vi "Load and Validate.vi"(8 "error in (no error)":errorcluster, 10 "Report Folder":path, 11 "Project Path":path) -> (0 "error out":errorcluster, 1 "Valid?":bool, 2 "Invalid Sections":string[](array[string]), 3 "Run cluster":T1)   [LabVIEW 2020, in "ProjectBuilder.lvlib" / "Project Builder.lvclass"]
uses:
  Project Builder.lvclass
  Ctl/Ctl_Run Cluster.ctl
  Action/Project Action/Project Action.lvclass
  Report Action/Report Action/Report Action.lvclass
  Ctl/Ctl_Build Steps.ctl
  Action/Project Action/Project Action.lvclass/Project Action.ctl
  PPL/HDH.ClassLoader.lvlibp
  <vilib>/Utility/config.llb/NI_LVConfig.lvlib
  ProjectBuilder.lvlib
  <vilib>/Utility/Data Type/NI_Data Type.lvlib
  Interface/Action Interface/Action Interface.lvclass
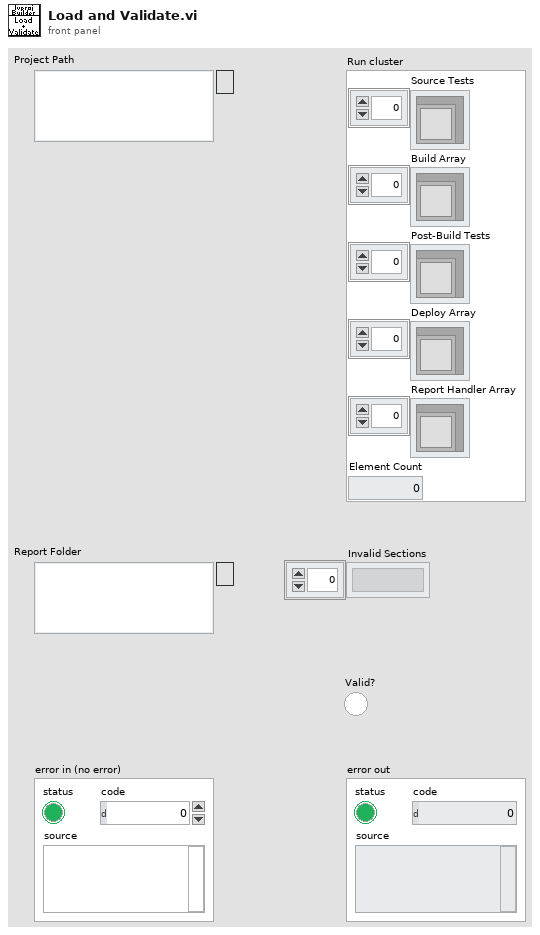
[diagram p1: front panel]
types:
  T1 = typedef "ProjectBuilder.lvlib/Project Builder.lvclass/Ctl_Run Cluster.ctl" = cluster{"Source Tests":refnum<class "Project Action.lvclass">[], "Build Array":refnum<class "Project Action.lvclass">[], "Post-Build Tests":refnum<class "Project Action.lvclass">[], "Deploy Array":refnum<class "Project Action.lvclass">[], "Report Handler Array":refnum<class "Report Action.lvclass">[], "Element Count":i32}
  T2 = typedef "ProjectBuilder.lvlib/Ctl_Build Steps.ctl" = enum16{"Source Test", "Build", "Post-Build Test", "Deploy", "Report"}
  T3 = typedef "NI_LVConfig.lvlib/Config Data RefNum.ctl" = refnum<k1>
  T4 = cluster{"Build Step":T2, "Last number":i32, "String":string}
  T5 = cluster{"Build Step":T2, "Last number":i32, "String":string}[]
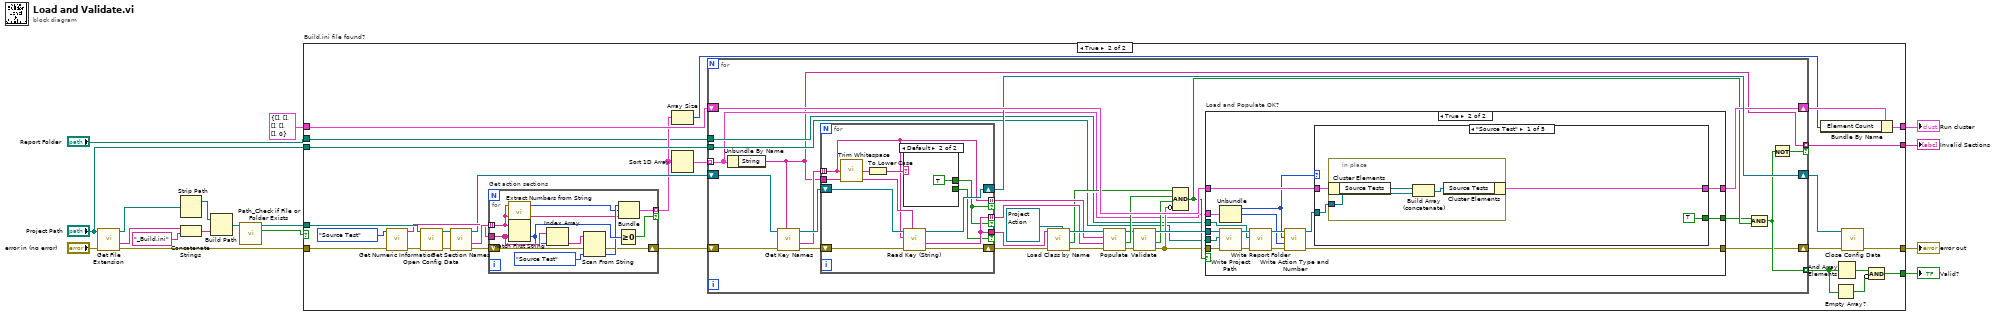
[diagram p0: block diagram]
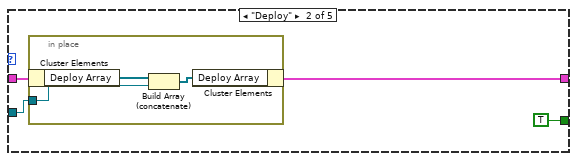
[diagram p4: hidden frame]
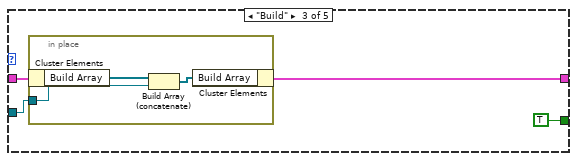
[diagram p5: hidden frame]
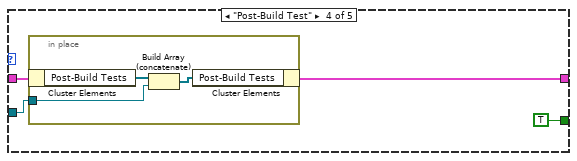
[diagram p6: hidden frame]
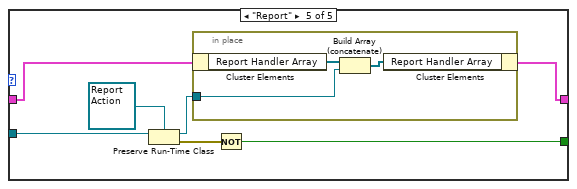
[diagram p7: hidden frame]
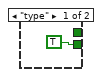
[diagram p8: hidden frame]
diagram:
  n1 = call <vilib>:"Get File Extension.vi"("error in (no error)"="error in (no error)", "file"="Project Path") -> ("error out"=w8:errorcluster, "filename without extension"=w17:string, "dup file"=w14:path)  [unwired: 5 in, 2 out]
  n2 = Strip Path(path=w14) -> (stripped path=w13:path)  [unwired: 1 out]
  n3 = Concatenate Strings(w17, "_Build.ini" ("string")) -> (w12:string)
  n4 = Build Path(base path=w13, name or relative path=w12) -> (appended path=w11:path)
  n5 = call "Path_Check if File or Folder Exists.vi"("File or Folder Path in"=w11) -> ("File or Folder Found?"=w10:bool, "File or Folder Path dub"=w9:path)  [unwired: 9 in]
  n6 = case "Build.ini file found?" shown="True" w10 {
    tunnel: w9 -> [_ w46]
    tunnel: w8 -> [w19 w40]
    tunnel: [w19 w37] -> w7
    tunnel: [w18 w25] -> w6
    tunnel: T1 {"Source Tests"=[], "Build Array"=[], "Post-Build Tests"=[], "Deploy Array"=[], "Report Handler Array"=[], "Element Count"=0} ("Run Cluster") -> [w18 w30]
    tunnel: [_ w21] -> w5
    tunnel: [_ w28] -> w4
    tunnel: "Project Path" -> [_ w27]
    tunnel: "Report Folder" -> [_ w23]
    frame False {
    }
    frame True {
      n7 = call <vilib>:"Get Numeric Information.vi"("error in (no error)"=w40, "variant"=Ctl_Build_Steps."Source Test" ("Build Step")) -> ("error out"=w39:errorcluster, "enum names"=w41:string[])  [unwired: 6 in, 2 out]
      n8 = call <vilib>:"Open Config Data.vi"("error in (no error)"=w39, "configuration file path"=w46) -> ("error out"=w44:errorcluster, "refnum"=w45:T3)  [unwired: 7 in, 1 out]
      n9 = call <vilib>:"Get Section Names.vi"("error in (no error)"=w44, "refnum"=w45) -> ("error out"=w38:errorcluster, "section names"=w43:string[], "refnum out"=w33:T3)  [unwired: 7 in]
      n10 = for "Get action sections" {
        tunnel: w43 -> [w147] mode=indexing
        tunnel: w41 -> [w157]
        shift-right: [w148] -> w35
        shift-left: w38 -> [w155]
        tunnel: [w154] -> w26 mode=indexing if=w153
        n11 = call "Extract Numbers from String.vi"("String"=w147) -> ("Last number"=w149:i32)  [unwired: 9 in, 1 out]
        n12 = Match First String(2:w157, 3:w147) -> (0:w156:i32)  [unwired: 1 out]
        n13 = Index Array(array=w157, index=w156) -> (element=w152:string)
        n14 = Scan From String(input string=w152, error in=w155, default 1=Ctl_Build_Steps."Source Test" ("Build Step")) -> (error out=w148:errorcluster, output 1=w150:T2)  [unwired: 2 in, 2 out]
        n15 = Greater Or Equal To 0?(x=w156) -> (x >= 0?=w153:bool)
        n16 = Bundle("Build Step"=w150, "Last number"=w149, "String"=w147) -> (w154:T4)  [unwired: 1 in]
      }
      n17 = Array Size(array=w26) -> (size(s)=w24:i32)
      n18 = Sort 1D Array(array=w26) -> (sorted array=w36:T5)
      n19 = for {
        tunnel: w36 -> [w48] mode=indexing
        shift-right: [w51] -> w34
        shift-left: w35 -> [w75]
        shift-right: [w73] -> w32
        shift-left: w33 -> [w76]
        shift-right: [w58] -> w31
        shift-left: w30 -> [w77]
        tunnel: [w56] -> w22 mode=indexing
        tunnel: [w47] -> w28 mode=indexing if=w59
        tunnel: w27 -> [w50]
        tunnel: w23 -> [w49]
        n20 = Unbundle By Name(w48) -> ("String"=w47:string)
        n21 = call <vilib>:"Get Key Names.vi"("section"=w47, "error in (no error)"=w75, "refnum"=w76) -> ("error out"=w72:errorcluster, "key names"=w71:string[], "refnum out"=w74:T3)  [unwired: 5 in, 1 out]
        n22 = for {
          shift-right: [w143] -> w73
          shift-left: w74 -> [w144]
          shift-right: [w141] -> w69
          shift-left: w72 -> [w142]
          tunnel: w71 -> [w134] mode=indexing
          tunnel: w47 -> [w140]
          tunnel: [w139] -> w64 mode=indexing if=w136
          tunnel: [w134] -> w65 mode=indexing if=w136
          tunnel: [w139] -> w70 if=w135
          n23 = call <vilib>:"Trim Whitespace.vi"("string"=w134) -> ("trimmed string"=w138:string)  [unwired: 1 in]
          n24 = To Lower Case(string=w138) -> (all lower case string=w137:string)
          n25 = case shown="Default" w137 {
            tunnel: [_ TRUE] -> w136
            tunnel: [TRUE _] -> w135
            frame "type" {
            }
            frame Default {
            }
          }
          n26 = call <vilib>:"Read Key (String).vi"("section"=w140, "error in (no error)"=w142, "key"=w134, "refnum"=w144) -> ("error out"=w141:errorcluster, "value"=w139:string, "refnum out"=w143:T3)  [unwired: 4 in, 1 out]
        }
        n27 = call "Load Class by Name.vi"("Class Type"=refnum<class "Project Action.lvclass"> refnum ("ProjectBuilder.lvlib:Project Action.lvclass"), "error in (no error)"=w69, "Base Class Name"=w70) -> ("error out"=w68:errorcluster, "Load and Type Success?"=w54:bool, "Loaded Class"=w66:refnum<class "Project Action.lvclass">)  [unwired: 5 in, 1 out]
        n28 = call "Populate.vi"("error in (no error)"=w68, "Values"=w64, "Names"=w65, "Action Interface in"=w66) -> ("error out"=w67:errorcluster, "Success?"=w63:bool, "Action Interface out"=w62:refnum<class "Project Action.lvclass">)  [unwired: 5 in]
        n29 = call "Validate.vi"("error in (no error)"=w67, "Action Interface in"=w62) -> ("error out"=w52:errorcluster, "Valid?"=w60:bool, "Action Interface out"=w61:refnum<class "Project Action.lvclass">)  [unwired: 7 in]
        n30 = Compound Arithmetic op=AND(w54, w63, w60, invert w52) -> (w57:bool)
        n31 = case "Load and Populate OK?" shown="True" w57 {
          tunnel: w77 -> [w79 w95]
          tunnel: w61 -> [_ w91]
          tunnel: [w79 w94] -> w58
          tunnel: [_ w93] -> w53
          tunnel: [w78 w89] -> w51
          tunnel: w52 -> [w78 w92]
          tunnel: w50 -> [_ w90]
          tunnel: w49 -> [_ w83]
          tunnel: w48 -> [_ w82]
          frame False {
          }
          frame True {
            n32 = Unbundle(w82) -> ("Build Step"=w80:T2, "Last number"=w81:i32)  [unwired: 1 out]
            n33 = call "Write Project Path.vi"("error in (no error)"=w92, "Project Path"=w90, "Project Action in"=w91) -> ("error out"=w85:errorcluster, "Project Action out"=w87:refnum<class "Project Action.lvclass">)  [unwired: 7 in]
            n34 = call "Write Report Folder.vi"("error in (no error)"=w85, "Report Folder"=w83, "Project Action in"=w87) -> ("error out"=w84:errorcluster, "Project Action out"=w86:refnum<class "Project Action.lvclass">)  [unwired: 7 in]
            n35 = call "Write Action Type and Number.vi"("error in (no error)"=w84, "Action Number"=w81, "Build Step"=w80, "Project Action in"=w86) -> ("error out"=w89:errorcluster, "Project Action out"=w88:refnum<class "Project Action.lvclass">)  [unwired: 6 in]
            n36 = case shown="\"Source Test\"" w80 {
              tunnel: w95 -> [w98 w106 w112 w119 w128]
              tunnel: w88 -> [w99 w104 w113 w120 w130]
              tunnel: [w97 w105 w111 w118 w126] -> w94
              tunnel: [TRUE TRUE TRUE TRUE w124] -> w93
              frame "Source Test" {
                n37 = in-place {
                  in-place-border: w99 -> [w101]
                  n38 = in-place-cluster #1(w98) -> ("Source Tests"=w102:refnum<class "Project Action.lvclass">[])
                  n39 = Build Array (concatenate)(w102, w101) -> (w100:refnum<class "Project Action.lvclass">[])
                  n40 = in-place-cluster #1("Source Tests"=w100) -> (w97:T1)
                }
              }
              frame "Deploy" {
                n41 = in-place {
                  in-place-border: w104 -> [w108]
                  n42 = in-place-cluster #2(w106) -> ("Deploy Array"=w109:refnum<class "Project Action.lvclass">[])
                  n43 = Build Array (concatenate)(w109, w108) -> (w107:refnum<class "Project Action.lvclass">[])
                  n44 = in-place-cluster #2("Deploy Array"=w107) -> (w105:T1)
                }
              }
              frame "Build" {
                n45 = in-place {
                  in-place-border: w113 -> [w115]
                  n46 = in-place-cluster #3(w112) -> ("Build Array"=w116:refnum<class "Project Action.lvclass">[])
                  n47 = Build Array (concatenate)(w116, w115) -> (w114:refnum<class "Project Action.lvclass">[])
                  n48 = in-place-cluster #3("Build Array"=w114) -> (w111:T1)
                }
              }
              frame "Post-Build Test" {
                n49 = in-place {
                  in-place-border: w120 -> [w122]
                  n50 = in-place-cluster #4(w119) -> ("Post-Build Tests"=w123:refnum<class "Project Action.lvclass">[])
                  n51 = Build Array (concatenate)(w123, w122) -> (w121:refnum<class "Project Action.lvclass">[])
                  n52 = in-place-cluster #4("Post-Build Tests"=w121) -> (w118:T1)
                }
              }
              frame "Report" {
                n53 = Preserve Run-Time Class(object in=w130, 2:refnum<class "Report Action.lvclass"> refnum ("ProjectBuilder.lvlib:Report Handler.lvclass")) -> (object out=w127:refnum<class "Report Action.lvclass">, error out=w125:errorcluster)  [unwired: 1 in]
                n54 = in-place {
                  in-place-border: w127 -> [w132]
                  n55 = in-place-cluster #5(w128) -> ("Report Handler Array"=w133:refnum<class "Report Action.lvclass">[])
                  n56 = Build Array (concatenate)(w133, w132) -> (w131:refnum<class "Report Action.lvclass">[])
                  n57 = in-place-cluster #5("Report Handler Array"=w131) -> (w126:T1)
                }
                n58 = Not(x=w125) -> (.not. x?=w124:bool)
              }
            }
          }
        }
        n59 = Compound Arithmetic op=AND(w53, w57) -> (w56:bool)
        n60 = Not(x=w56) -> (.not. x?=w59:bool)
      }
      n61 = Bundle By Name(cluster=w31, "Element Count"=w24) -> (w25:T1)
      n62 = Empty Array?(array=w22) -> (empty?=w20:bool)
      n63 = And Array Elements(Boolean array=w22) -> (logical AND=w29:bool)
      n64 = call <vilib>:"Close Config Data.vi"("error in (no error)"=w34, "refnum"=w32) -> ("error out"=w37:errorcluster)  [unwired: 8 in, 1 out]
      n65 = Compound Arithmetic op=AND(w29, invert w20) -> (w21:bool)
    }
  }
  "error out" <- w7
  "Run cluster" <- w6
  "Valid?" <- w5
  "Invalid Sections" <- w4
